vi "close.vi"(8 "error in (no error)":errorcluster, 11 "Logger in":refnum<class "Logger.lvclass">) -> (0 "error out":errorcluster, 2 "filePathClosed":path, 3 "Logger out":refnum<class "Logger.lvclass">)   [LabVIEW 2018, in "Logger.lvclass"]
doc: "Close the log file."
uses:
  Logger.lvclass
  Logger.lvclass/Logger.ctl
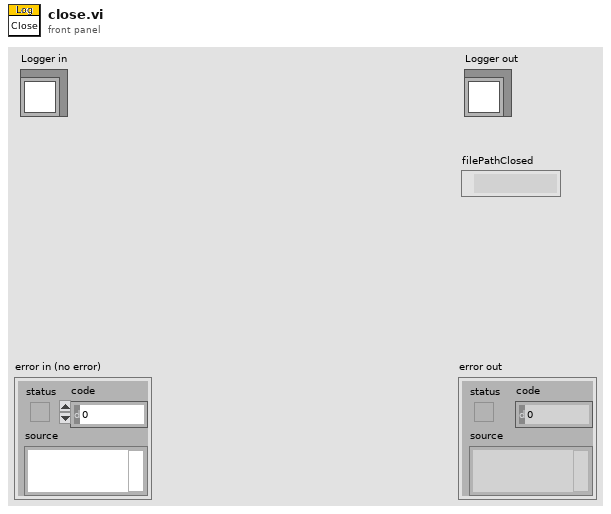
[diagram p1: front panel]
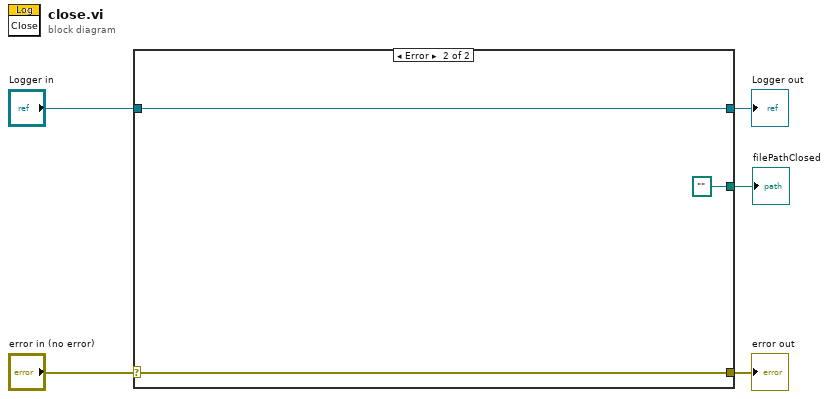
[diagram p0: block diagram]
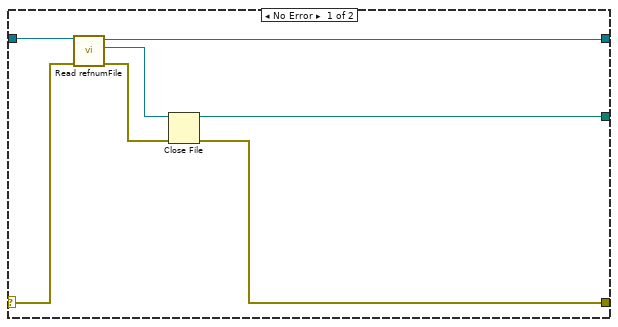
[diagram p2: hidden frame]
diagram:
  n1 = case shown="Error" "error in (no error)" {
    selector: "error in (no error)" -> [w10 w15]
    tunnel: [w7 w15] -> w4
    tunnel: [w11 w14] -> w2
    tunnel: "Logger in" -> [w12 w14]
    tunnel: [w6 path "" ("path")] -> w1
    frame No Error {
      n2 = call "Read refnumFile.vi"("error in (no error)"=w10, "Logger in"=w12) -> ("error out"=w8:errorcluster, "refnumFile"=w9:refnum<file>, "Logger out"=w11:refnum<class "Logger.lvclass">)  [unwired: 7 in]
      n3 = Close File(refnum=w9, error in=w8) -> (path=w6:path, error out=w7:errorcluster)
    }
    frame Error {
    }
  }
  "error out" <- w4
  "Logger out" <- w2
  "filePathClosed" <- w1
